vi "Get Trailing Arguments.vi"(8 "error in (no error)":errorcluster, 11 "Option Set in":refnum<class "Option Set.lvclass">) -> (0 "error out":errorcluster, 2 "Arguments":string[](array[string]), 3 "Option Set out":refnum<class "Option Set.lvclass">)   [LabVIEW 2011, in "Option Parser.lvlib" / "Option Set.lvclass"]
doc: "Gets any arguments that were attached to an option set by the user."
uses:
  Option Set.lvclass
  Option Set.lvclass/Option Set.ctl
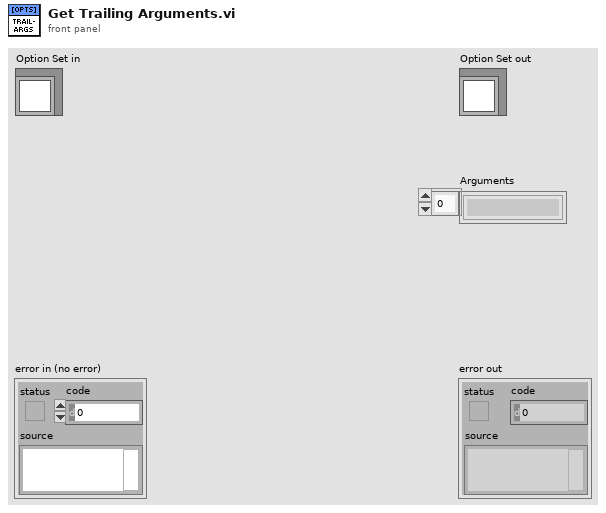
[diagram p1: front panel]
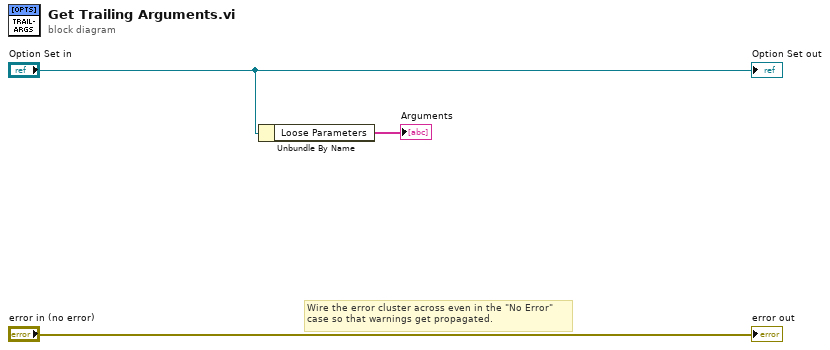
[diagram p0: block diagram]
diagram:
  # "Wire the error cluster across even in the \"No Error\"\ncase so that warnings get propagated."
  n1 = Unbundle By Name("Option Set in") -> ("Loose Parameters"=→"Arguments":string[])
  "error out" <- "error in (no error)"
  "Option Set out" <- "Option Set in"
